vi "test ws client.vi"() -> ()   [LabVIEW 2016]
uses:
  websocket/client/websocket client.lvclass
panel:
  out "lens":i32
  out "lenr":i32
  out "error out 2":errorcluster
  in  "send bin":bool
  in  "send txt":bool
  in  "DATA to send":string
  out "op":u8=2
  out "message":string
  out "final messages":string[](array[string])
  in  "stop":bool
  out "error out":errorcluster
  in  "address":string="localhost"
  in  "port":u16=8095
  in  "url":string="dsfs"
  in  "error in":errorcluster
  in  "host header":string="sdfs"
  in  "subprotocols":string[](array[string])=["sdfs"]
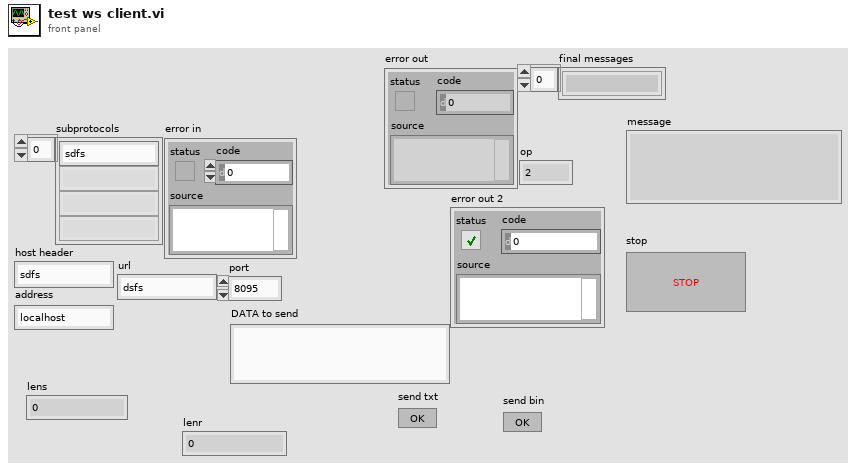
[diagram p1: front panel]
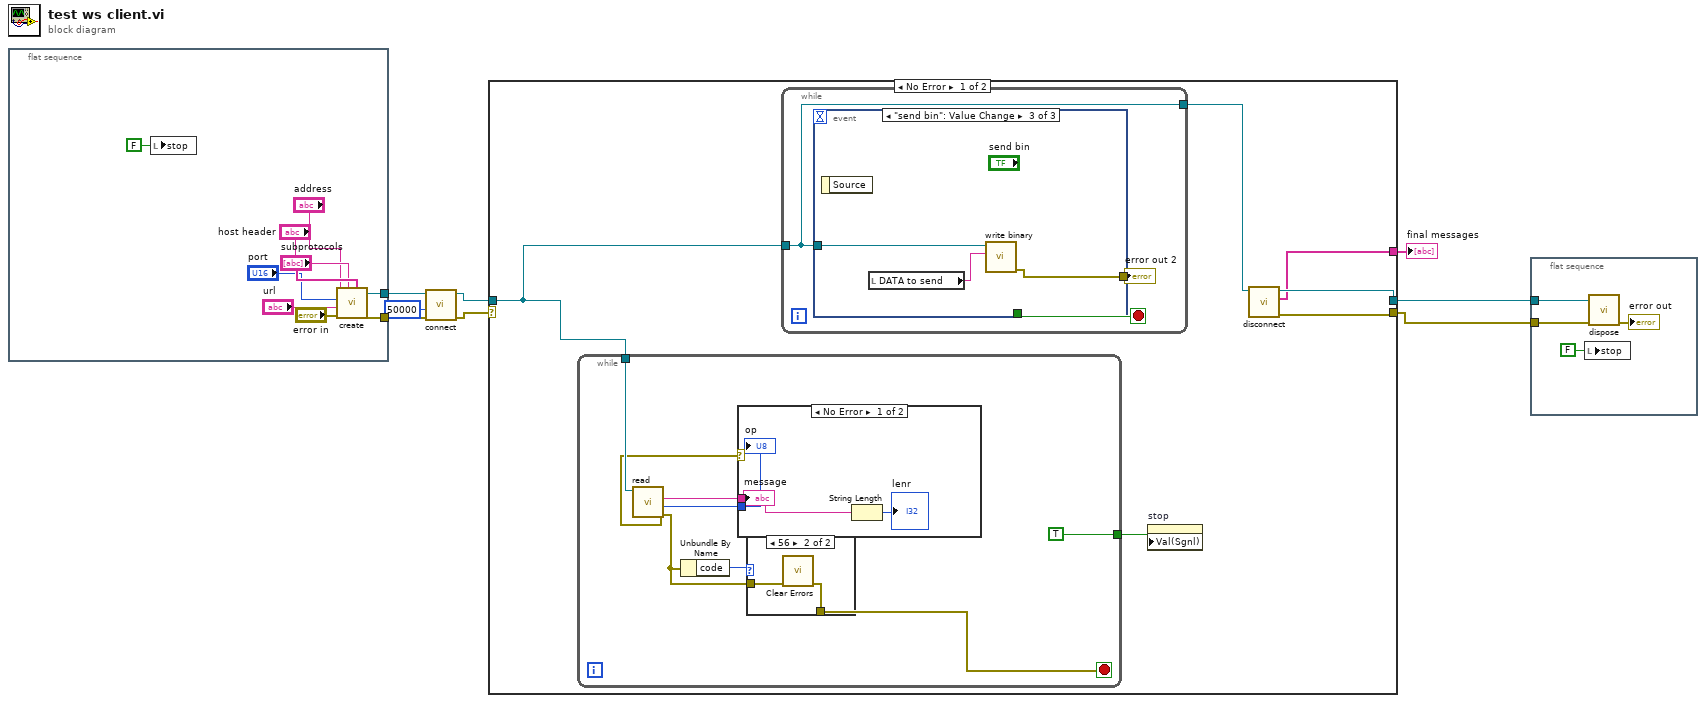
[diagram p0: block diagram]
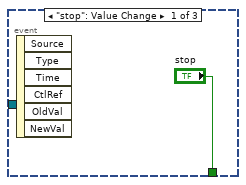
[diagram p2: hidden frame]
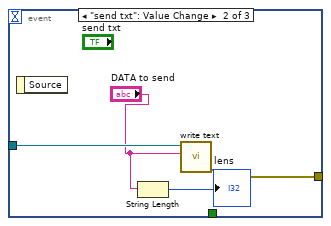
[diagram p3: hidden frame]
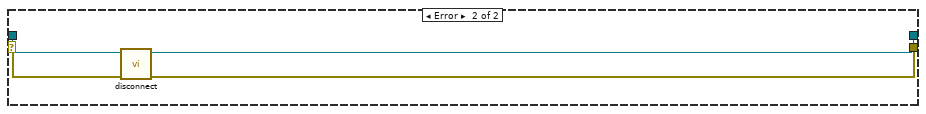
[diagram p6: hidden frame]
diagram:
  n1 = flat-sequence {
    tunnel: [w17] -> w8
    tunnel: [w16] -> w7
    frame #0 {
      n2 = local write "stop"(FALSE ("stop")) -> ()
      n3 = call "create.vi"("subprotocols"="subprotocols", "host header"="host header", "error in"="error in", "url"="url", "port"="port", "address"="address") -> ("error out"=w16:errorcluster, "websocket client out"=w17:refnum<class "websocket client.lvclass">)  [unwired: 4 in]
    }
  }
  n4 = call "connect.vi"("error in"=w7, "timeout ms (5000)"=50000, "websocket client in"=w8) -> ("error out"=w6:errorcluster, "websocket client out"=w5:refnum<class "websocket client.lvclass">)  [unwired: 7 in]
  n5 = case shown="No Error" w6 {
    selector: w6 -> [_ w51]
    tunnel: [w22 w48] -> w4
    tunnel: w5 -> [w19 w50]
    tunnel: [w23 w49] -> w3
    tunnel: [w21 _] -> w2
    frame No Error {
      n6 = while {
        tunnel: w19 -> [w41]
        tunnel: [TRUE ("Value (Signaling)")] -> w20
        stop <- w38 stop-if-true
        n7 = call "read.vi"("websocket client in"=w41) -> ("error out"=w36:errorcluster, "Numeric"=w37:u8, "message"=w39:string)  [unwired: 7 in, 1 out]
        n8 = Unbundle By Name(w36) -> ("code"=w35:i32)
        n9 = case shown="No Error" w36 {
          tunnel: w39 -> [w46 _]
          tunnel: w37 -> [w47 _]
          frame No Error {
            n10 = String Length(string=w46) -> (length=→"lenr":i32)
            "message" <- w46
            "op" <- w47
          }
          frame Error {
          }
        }
        n11 = case shown="56" w35 {
          tunnel: [w42 w44] -> w38
          tunnel: w36 -> [w42 w43]
          frame 0, Default {
          }
          frame 56 {
            n12 = call <vilib>:"Clear Errors.vi"("error in (no error)"=w43) -> ("error out"=w44:errorcluster)  [unwired: 5 in, 1 out]
          }
        }
      }
      n13 = while {
        tunnel: w19 -> [w24]
        tunnel: [w24] -> w18
        stop <- w26 stop-if-true
        n14 = event shown="[2] \"send bin\": Value Change" {
          selector: _ -> [_ _ _]
          dyn-events: _ -> [_ _ _]
          timeout: _ -> [_ _ _]
          tunnel: ["stop" _ _] -> w26
          tunnel: w24 -> [_ w31 w34]
          tunnel: [_ w30 w33] -> w25
          event "stop": Value Change {
            n15 = event-data() -> ()  [unwired: 1 in, 6 out]
          }
          event "send txt": Value Change {
            n16 = event-data() -> ()  [unwired: 1 in, 1 out]
            n17 = String Length(string="DATA to send") -> (length=→"lens":i32)
            n18 = call "write text.vi"("text"="DATA to send", "websocket client in"=w31) -> ("error out"=w30:errorcluster)  [unwired: 8 in, 1 out]
          }
          event "send bin": Value Change {
            n19 = event-data() -> ()  [unwired: 1 in, 1 out]
            n20 = local read "DATA to send"() -> (w32:string)
            n21 = call "write binary.vi"("binary"=w32, "websocket client in"=w34) -> ("error out"=w33:errorcluster)  [unwired: 8 in, 1 out]
          }
        }
        "error out 2" <- w25
      }
      n22 = property on="stop" class="Bool (strict)"("Val(Sgnl)"=w20) -> ()  [unwired: 2 in, 2 out]
      n23 = call "disconnect.vi"("websocket client in"=w18) -> ("error out"=w23:errorcluster, "final messages"=w21:string[], "websocket client out"=w22:refnum<class "websocket client.lvclass">)  [unwired: 8 in]
    }
    frame Error {
      n24 = call "disconnect.vi"("error in"=w51, "websocket client in"=w50) -> ("error out"=w49:errorcluster, "websocket client out"=w48:refnum<class "websocket client.lvclass">)  [unwired: 7 in, 1 out]
    }
  }
  "final messages" <- w2
  n25 = flat-sequence {
    tunnel: w4 -> [w55]
    tunnel: w3 -> [w54]
    frame #0 {
      n26 = local write "stop"(FALSE ("stop")) -> ()
      n27 = call "dispose.vi"("error in"=w54, "websocket client in"=w55) -> ("error out"=→"error out":errorcluster)  [unwired: 9 in]
    }
  }
